vi "Shift right.vi"(0 "Num In":u16 format="%.0x") -> (1 "Num Out":u16 format="%.0x", 2 "LSB":bool)   [LabVIEW 2009]
panel:
  out "in array":bool[](array[boolean])
  out "output array":bool[](array[boolean])
  # "LSB Shift right and Cut,\n to MSB add 0"
  # "D0"
  # "D15"
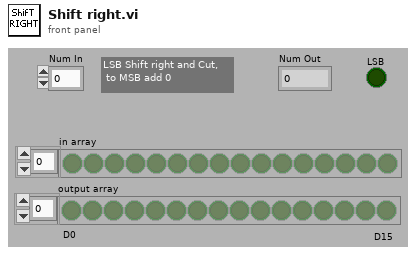
[diagram p1: front panel]
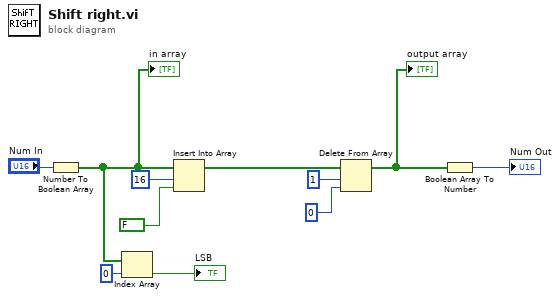
[diagram p0: block diagram]
diagram:
  n1 = Number To Boolean Array(number="Num In") -> (Boolean array=w3:bool[])
  "in array" <- w3
  n2 = Index Array(array=w3, index=0) -> (element=→"LSB":bool)
  n3 = Insert Into Array "Insert Into Array"(array=w3, index=16, new element=FALSE ("new element/subarray")) -> (w6:bool[])
  n4 = Delete From Array "Delete From Array"(array=w6, length=1, index=0) -> (array with subset deleted=w5:bool[])  [unwired: 1 out]
  "output array" <- w5
  n5 = Boolean Array To Number(Boolean array=w5) -> (number=→"Num Out":u32)
